vi "TDS_ErrorHandler.vi"(8 "error in":errorcluster, 11 "VI ServerCluster":T1) -> (0 "error out":errorcluster, 3 "VI ServerCluster DUP":T1)   [LabVIEW 2020]
uses:
  LabVIEW 2020 Toolkits/VI Server Toolkit/VI Server_TypeDefs/VI Server_RefsCluster.ctl
  LabVIEW 2020 Toolkits/VI Server Toolkit/VI Server Libraries/VI Server_Set Controls.llb/Set STR Control.vi
  LabVIEW 2020 Toolkits/VI Server Toolkit/VI Server Toolkit LV2013.lvlib
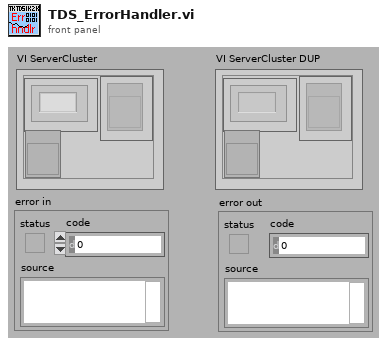
[diagram p1: front panel]
types:
  T1 = typedef "VI Server_RefsCluster.ctl" = cluster{"Labels":string[], "Refs":refnum<vi>[], "VI Ref":refnum<vi>}
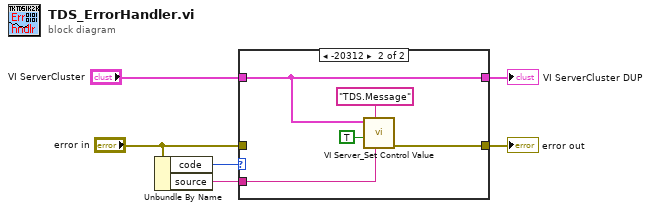
[diagram p0: block diagram]
diagram:
  n1 = Unbundle By Name("error in") -> ("code"=w4:i32, "source"=w2:string)
  n2 = case shown="-20312" w4 {
    tunnel: "error in" -> [w8 _]
    tunnel: [w8 w13] -> w6
    tunnel: "VI ServerCluster" -> [w7 w10]
    tunnel: w2 -> [_ w12]
    tunnel: [w7 w10] -> w1
    frame 0, Default {
    }
    frame -20312 {
      n3 = call-poly "VI Server_Set Control Value.vi"("New Value"=w12, "Label"="TDS.Message", "Single Instance (T)"=TRUE, "VI Server Cluster"=w10) -> ("error out"=w13:errorcluster)  [unwired: 5 in, 2 out]
    }
  }
  "error out" <- w6
  "VI ServerCluster DUP" <- w1
